vi "层叠式顺序结构.vi"() -> ()   [LabVIEW 2022 SP3]
doc: "本VI是为《我和LabVIEW》一书编写的示例。\n关于本书的介绍请参考网页：\nhttp://ruanqizhen.spaces.live.com/blog/cns!5852D4F797C53FB6!4310.entry"
panel:
  out "程序耗时":dbl caption="Time to Match" format="%.3f"
  out "迭代次数":i32=124 caption="# of iterations"
  out "当前数值":i32=5 caption="Current Number"
  in  "比较数值":i32=123 min=0 max=100000 step=1
  # "sec"
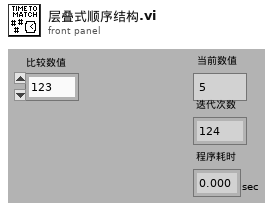
[diagram p1: front panel]
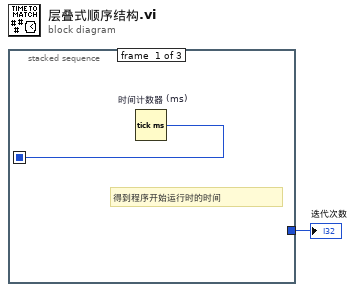
[diagram p0: block diagram]
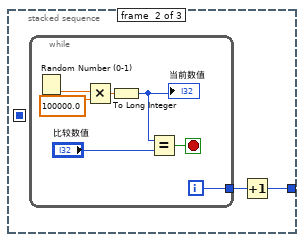
[diagram p2: hidden frame]
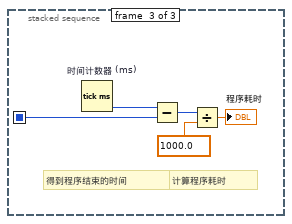
[diagram p3: hidden frame]
diagram:
  n1 = stacked-sequence {
    seq-local: [w2 _ _] -> [_ _ w12]
    tunnel: [_ w3 _] -> w1
    frame #0 {
      # "得到程序开始运行时的时间"
      n2 = Tick Count (ms) "时间计数器 (ms)"() -> (millisecond timer value=w2:u32)
    }
    frame #1 {
      n3 = while {
        tunnel: [w6] -> w4
        i -> [w6]
        stop <- w7 stop-if-true
        n4 = Random Number (0-1)() -> (number: 0 to 1=w11:dbl)
        n5 = Multiply(x=w11, y=100000.0) -> (x*y=w9:dbl)
        n6 = To Long Integer(number=w9) -> (32bit integer=w5:i32)
        "当前数值" <- w5
        n7 = Equal?(x=w5, y="比较数值") -> (x = y?=w7:bool)
      }
      n8 = Increment(x=w4) -> (x+1=w3:i32)
    }
    frame #2 {
      # "计算程序耗时"
      # "得到程序结束的时间"
      n9 = Tick Count (ms) "时间计数器 (ms)"() -> (millisecond timer value=w16:u32)
      n10 = Subtract(x=w16, y=w12) -> (x-y=w15:u32)
      n11 = Divide(x=w15, y=1000.0) -> (x/y=→"程序耗时":dbl)
    }
  }
  "迭代次数" <- w1
